vi "Mandelbrot_generatorNT.vi"() -> ()   [LabVIEW 2015]
panel:
  in  "React VI":u16(ring) items=["", "Rworker.vi"]
  in  "Async ?":bool
  in  "machine name (\"\":  open local reference)":string
  in  "Cicli":i32=200
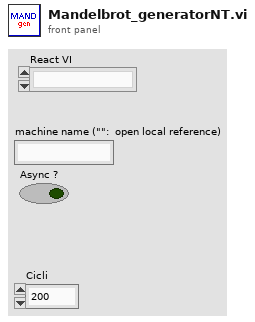
[diagram p1: front panel]
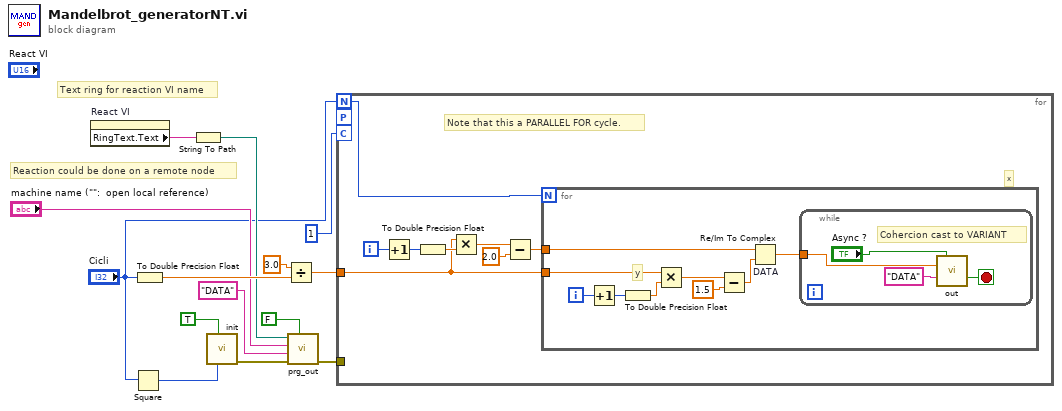
[diagram p0: block diagram]
diagram:
  # "Text ring for reaction VI name"
  # "Reaction could be done on a remote node"
  n1 = property on="React VI" class="Ring (strict)"() -> ("RingText.Text"=w1:string)  [unwired: 2 in, 2 out]
  n2 = Square(x="Cicli") -> (x^2=w3:i32)
  n3 = To Double Precision Float(number="Cicli") -> (double precision float=w9:dbl)
  n4 = String To Path(string=w1) -> (path=w8:path)
  n5 = call "init.vi"("Space size"=w3, "Cleaneup"=TRUE ("Cleneup")) -> ("error out"=w5:errorcluster)  [unwired: 9 in]
  n6 = Divide(x=3.0, y=w9) -> (x/y=w13:dbl)
  n7 = call "prg_out.vi"("Reset to default"=FALSE, "error in (no error)"=w5, "Name"="DATA" ("String"), "machine name (\"\":  open local reference)"="machine name (\"\":  open local reference)", "vi path"=w8) -> ("error out"=w11:errorcluster)  [unwired: 6 in]
  n8 = for {
    N: "Cicli" -> [w15]
    tunnel: w13 -> [w21]
    tunnel: w11 -> [_]
    workers-P: _ -> [_]
    chunk-C: 1 -> [_]
    i -> [w19]
    # "Note that this a PARALLEL FOR cycle."
    # "x"
    n9 = Increment(x=w19) -> (x+1=w16:i32)
    n10 = To Double Precision Float(number=w16) -> (double precision float=w22:dbl)
    n11 = Multiply(x=w21, y=w22) -> (x*y=w17:dbl)
    n12 = Subtract(x=w17, y=2.0) -> (x-y=w20:dbl)
    n13 = for {
      N: w15 -> [_]
      tunnel: w21 -> [w30]
      tunnel: w20 -> [w27]
      i -> [w25]
      # "y"
      n14 = Increment(x=w25) -> (x+1=w24:i32)
      n15 = To Double Precision Float(number=w24) -> (double precision float=w31:dbl)
      n16 = Multiply(x=w30, y=w31) -> (x*y=w29:dbl)
      n17 = Subtract(x=w29, y=1.5) -> (x-y=w26:dbl)
      n18 = Re/Im To Complex "DATA"(1:w26, 2:w27) -> (0:w23:cdb)
      n19 = while {
        tunnel: w23 -> [w35]
        stop <- w34 stop-if-true
        # "Cohercion cast to VARIANT"
        n20 = call "out.vi"("Async ?"="Async ?", "IN VARIANT"=w35, "Name in"="DATA" ("Name out")) -> ("Operation Ok"=w34:bool)  [unwired: 11 in, 1 out]
      }
    }
  }
